vi "Aliasing 2.vi"() -> ()   [LabVIEW 2016]
panel:
  out "Waveform Graph":waveform(dbl)[](graph)=[{"t0"=timestamp(0 s since 1904-01-01), "dt"=0.005, "Y"=array[400 elements]}, {"t0"=timestamp(0 s since 1904-01-01), "dt"=0.25, "Y"=[0.7071067811865476, -0.7071067811865475, -0.7071067811865477, 0.7071067811865474, 0.7071067811865477, -0.7071067811865467, -0.7071067811865471, 0.7071067811865466]}, {"t0"=timestamp(0 s since 1904-01-01), "dt"=0.005, "Y"=array[400 elements]}, {"t0"=timestamp(0 s since 1904-01-01), "dt"=0.005, "Y"=array[400 elements]}]
  in  "Tab Control":enum32{"Hovedside", "Innstillinger"}(tab)
  in  "fk color":u32(colorbox)=16777224
  in  "fm color":u32(colorbox)=16711680
  in  "f0 color":u32(colorbox)=16448250
  in  "f0":dbl=1.0
  in  "fs":dbl=4.0
  in  "l":i32
  out "f0 + l fs":dbl=1.0
  out "-f0 + m fs":dbl=-1.0
  in  "stop":bool
  in  "m":i32
  in  "Fase [Grader]":dbl=45.0
  in  "Perioder":i32=2
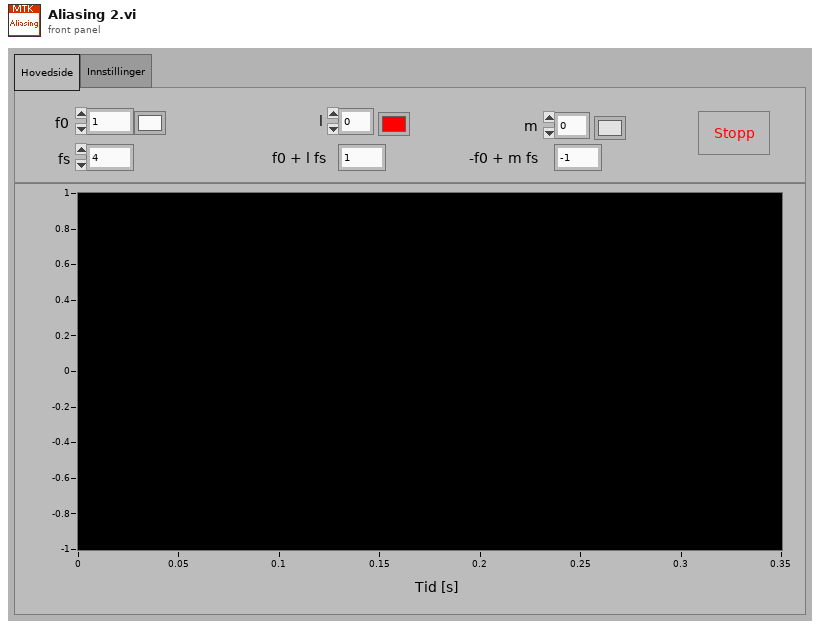
[diagram p1: front panel]
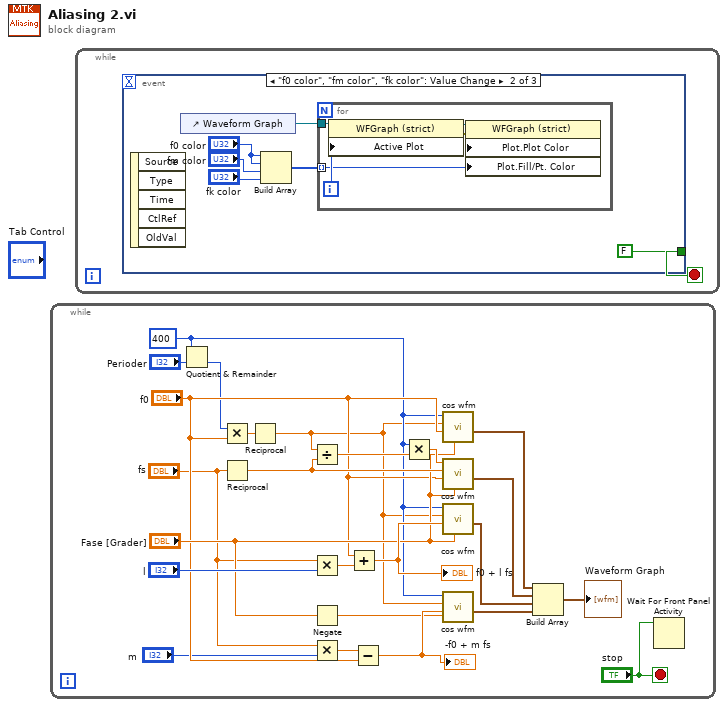
[diagram p0: block diagram]
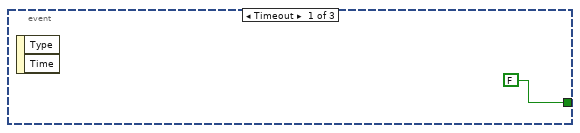
[diagram p2: hidden frame]
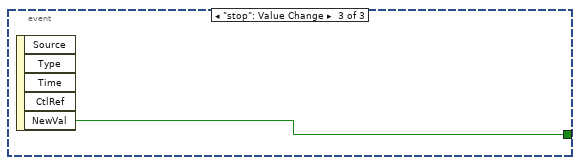
[diagram p3: hidden frame]
diagram:
  n1 = while {
    stop <- "stop" stop-if-true
    w11 = 400 ("samples")
    n2 = Quotient & Remainder(x=w11, y="Perioder") -> (floor(x/y)=w9:i32)  [unwired: 1 out]
    n3 = Multiply(x=w9, y="f0") -> (x*y=w13:dbl)
    n4 = Reciprocal(x="fs") -> (1/x=w20:dbl)
    n5 = Reciprocal(x=w13) -> (1/x=w8:dbl)
    n6 = Divide(x=w8, y=w20) -> (x/y=w19:dbl)
    n7 = Multiply(x="fs", y="l") -> (x*y=w6:dbl)
    n8 = Negate(x="Fase [Grader]") -> (-x=w14:dbl)
    n9 = Multiply(x="fs", y="m") -> (x*y=w7:dbl)
    n10 = Add(x="f0", y=w6) -> (x+y=w17:dbl)
    "f0 + l fs" <- w17
    n11 = Subtract(x=w7, y="f0") -> (x-y=w16:dbl)
    "-f0 + m fs" <- w16
    n12 = Multiply(x=w11, y=w19) -> (x*y=w18:dbl)
    n13 = call "cos wfm.vi"("phi"="Fase [Grader]", "f"="f0", "dt"=w8, "N"=w11) -> ("cos wt"=w23:waveform(dbl))  [unwired: 7 out]
    n14 = call "cos wfm.vi"("phi"="Fase [Grader]", "f"="f0", "dt"=w20, "N"=w18) -> ("cos wt"=w21:waveform(dbl))  [unwired: 7 out]
    n15 = call "cos wfm.vi"("phi"="Fase [Grader]", "f"=w17, "dt"=w8, "N"=w11) -> ("cos wt"=w3:waveform(dbl))  [unwired: 7 out]
    n16 = call "cos wfm.vi"("phi"=w14, "f"=w16, "dt"=w8, "N"=w11) -> ("cos wt"=w2:waveform(dbl))  [unwired: 7 out]
    n17 = Build Array(w23, w21, w3, w2) -> (→"Waveform Graph":waveform(dbl)[])
    n18 = Wait For Front Panel Activity(3:"stop") -> ()  [unwired: 3 out]
  }
  n19 = while {
    stop <- w25 stop-if-true
    n20 = event shown="[1] \"f0 color\", \"fm color\", \"fk color\": Value Change" {
      selector: _ -> [_ _ _]
      dyn-events: _ -> [_ _ _]
      timeout: _ -> [_ _ _]
      tunnel: [FALSE ("NewVal") FALSE ("NewVal") w38] -> w25
      event Timeout {
        n21 = event-data() -> ()  [unwired: 3 out]
      }
      event "f0 color", "fm color", "fk color": Value Change {
        n22 = event-data() -> ()  [unwired: 6 out]
        n23 = control-ref of="Waveform Graph"() -> (w28:refnum<vi>)
        n24 = Build Array("f0 color", "f0 color", "fm color", "fk color") -> (w29:u32[])
        n25 = for {
          tunnel: w29 -> [w33] mode=indexing
          tunnel: w28 -> [w37]
          i -> [w34]
          n26 = property class="WFGraph (strict)"(reference=w37, "Active Plot"=w34) -> (reference out=w36:refnum<vi>, error out=w35:errorcluster)  [unwired: 1 in]
          n27 = property class="WFGraph (strict)"(reference=w36, error in=w35, "Plot.Plot Color"=w33, "Plot.Fill/Pt. Color"=w33) -> ()  [unwired: 2 out]
        }
      }
      event "stop": Value Change {
        n28 = event-data() -> ("NewVal"=w38:bool)  [unwired: 5 out]
      }
    }
  }
